vi "Creat NewNode.vi"(8 "error in (no error)":errorcluster caption="错误输入（无错误）", 11 "PanelDataNode 输入":refnum<class "PanelDataNode.lvclass"> caption="DNL_LabVIEW Object in") -> (0 "error out":errorcluster caption="错误输出", 2 "NewNode*":refnum<data-value>, 3 "PanelDataNode 输出":refnum<class "PanelDataNode.lvclass"> caption="DNL_LabVIEW Object out")   [LabVIEW 2013, in "PanelDataNode.lvclass"]
uses:
  PanelDataNode.lvclass
  PanelLinkNode/PanelLinkNode.lvclass
  PanelDataNode.lvclass/PanelDataNode.ctl
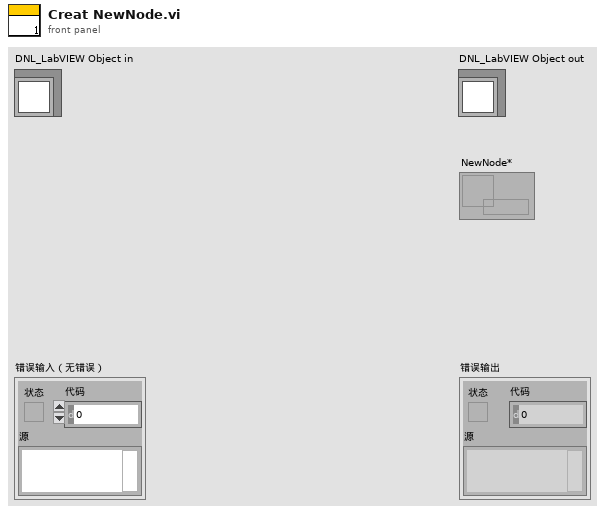
[diagram p1: front panel]
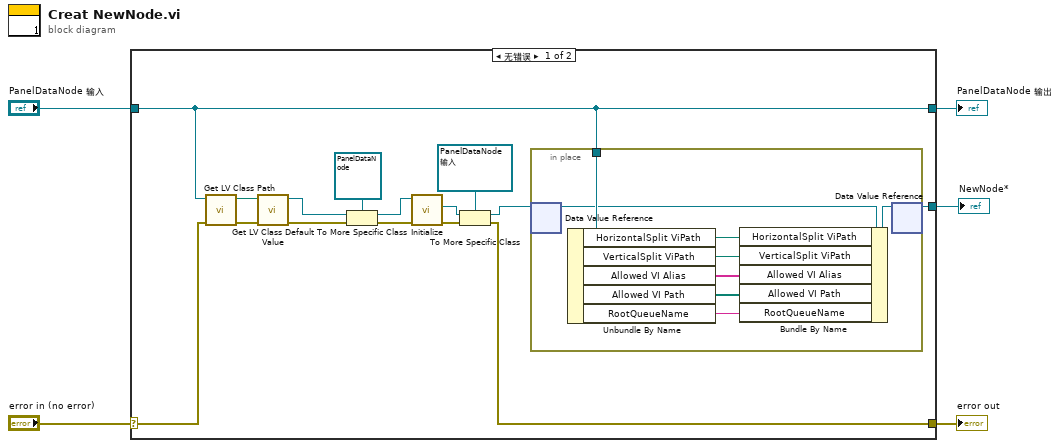
[diagram p0: block diagram]
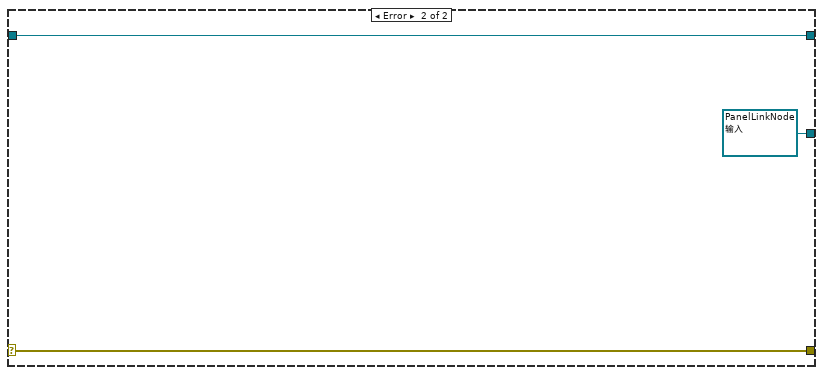
[diagram p2: hidden frame]
diagram:
  n1 = case shown="无错误" "error in (no error)" {
    selector: "error in (no error)" -> [w14 w31]
    tunnel: [w6 w31] -> w4
    tunnel: [w8 w30] -> w2
    tunnel: "PanelDataNode 输入" -> [w8 w30]
    tunnel: [w12 refnum<data-value> refnum ("SelfNode*")] -> w1
    frame No Error {
      n2 = call <vilib>:"Get LV Class Path.vi"("error in (no error)"=w14, "object"=w8) -> ("error out"=w18:errorcluster, "class path"=w15:path)  [unwired: 8 in]
      n3 = call <vilib>:"Get LV Class Default Value.vi"("error in (no error)"=w18, "class path"=w15) -> ("error out"=w20:errorcluster, "object"=w17:refnum<class>)  [unwired: 8 in]
      n4 = To More Specific Class(target class=refnum<class "PanelDataNode.lvclass"> refnum ("PanelDataNode.lvclass"), reference=w17, error in=w20) -> (specific class reference=w13:refnum<class "PanelDataNode.lvclass">, error out=w19:errorcluster)
      n5 = call-dynamic "Initialize.vi"("error in"=w19, "PanelDataNode in"=w13) -> ("error out"=w11:errorcluster, "SelfNode*"=w10:refnum<data-value>)  [unwired: 7 in]
      n6 = To More Specific Class(target class=refnum<data-value> refnum ("数据值引用"), reference=w10, error in=w11) -> (specific class reference=w9:refnum<data-value>, error out=w6:errorcluster)
      n7 = in-place {
        in-place-border: w8 -> [w28]
        n8 = in-place-dvr #1(w9) -> (w27:refnum<class "PanelDataNode.lvclass">)  [unwired: 1 out]
        n9 = Unbundle By Name(w28) -> ("HorizontalSplit ViPath"=w25:path, "VerticalSplit ViPath"=w24:path, "Allowed VI Alias"=w23:string[], "Allowed VI Path"=w22:path[], "RootQueueName"=w21:string)
        n10 = Bundle By Name(cluster=w27, "HorizontalSplit ViPath"=w25, "VerticalSplit ViPath"=w24, "Allowed VI Alias"=w23, "Allowed VI Path"=w22, "RootQueueName"=w21) -> (w26:refnum<class "PanelDataNode.lvclass">)
        n11 = in-place-dvr #1(w26) -> (w12:refnum<data-value>)  [unwired: 1 out]
      }
    }
    frame Error {
    }
  }
  "error out" <- w4
  "PanelDataNode 输出" <- w2
  "NewNode*" <- w1
